vi "RT 10Hz test 1.vi"() -> ()   [LabVIEW 2014]
uses:
  <vilib>/Platform/TimedLoop/XDataNode/timing_clust.ctl
  <vilib>/Platform/TimedLoop/XDataNode/nitl_modes.ctl
  <vilib>/Platform/TimedLoop/XDataNode/wakeup.ctl
  <vilib>/FPGAPlugInAG/cRIO-9067/niLvFpga_Open_cRIO-9067.vi
  <vilib>/Utility/error.llb/Error Cluster From Error Code.vi
  <vilib>/rvi/errors/niLvFpgaAdjustHostInterfaceError.vi
  <vilib>/FPGAPlugInAG/cRIO-9067/niLvFpga_Close_cRIO-9067.vi
  <vilib>/rvi/interface/nirviOpenFPGA/nirviOpenFPGA.xnode
  FPGA Bitfiles/MAXCAT_FPGATarget5_FPGAmainv06_iLwI+xiZeAU.lvbitx
  FPGA main v06.vi
  <vilib>/Platform/TimedLoop/XDataNode/XDataNode.xnode
  <vilib>/rvi/interface/nirviReadWriteControl/nirviReadWriteControl.xnode
  <vilib>/rvi/interface/nirviCloseFPGA/nirviCloseFPGA.xnode
  NiFpgaLv.dll
  <vilib>/Platform/TimedLoop/XDataNode/XDNodeRunTimeDep.lvlib
panel:
  out "Period 2":u32
  out "Period":u32
  out "Array 1 In":fxp<+/-,35,9>[](array[numeric])
  out "Array 2 In":fxp<+/-,30,9>[](array[numeric])
  in  "stop":bool
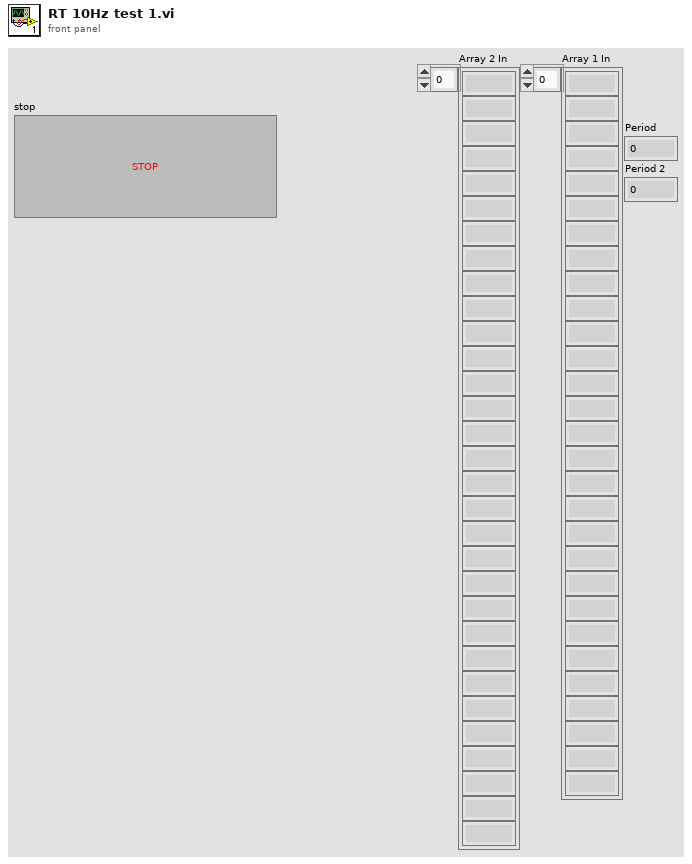
[diagram p1: front panel]
types:
  T1 = typedef "XDNodeRunTimeDep.lvlib/timing_clust.ctl" = cluster{"Expected End [f-1]":u64, "Actual End [f-1]":u64, "Finished Late? [f-1]":bool, "Expected End [i-1]":u64, "Actual End [i-1]":u64, "Finished Late? [i-1]":bool, "Expected Start [i]":u64, "Actual Start [i]":u64, "Expected Start [f]":u64, "Actual Start [f]":u64, "Source Name":string, "Structure Name":string, "Period":i64, "Deadline":i64, "Offset":i64, "Start":i64, "Priority":i32, "Timeout":i32, "Mode":T2, "Wakeup Reason":T3, "Error":errorcluster, "Source Type":string, "Secondary Source Type":string, "Global End Time":u64, "Global Start Time":u64, "Frame Duration":u64, "Iteration Duration":u64, "Assigned CPU":i32, "I/O Scan Engine Mode":u32}
  T2 = typedef "XDNodeRunTimeDep.lvlib/nitl_modes.ctl" = enum32{"No Change", "Process missed periods, maintain original phase", "Discard missed periods, maintain original phase", "Process missed periods, ignore original phase", "Discard missed periods, ignore original phase"}
  T3 = typedef "XDNodeRunTimeDep.lvlib/wakeup.ctl" = enum32{"Normal", "Aborted", "Asynchronous wakeup", "Timing source error", "Timed loop error", "Timeout"}
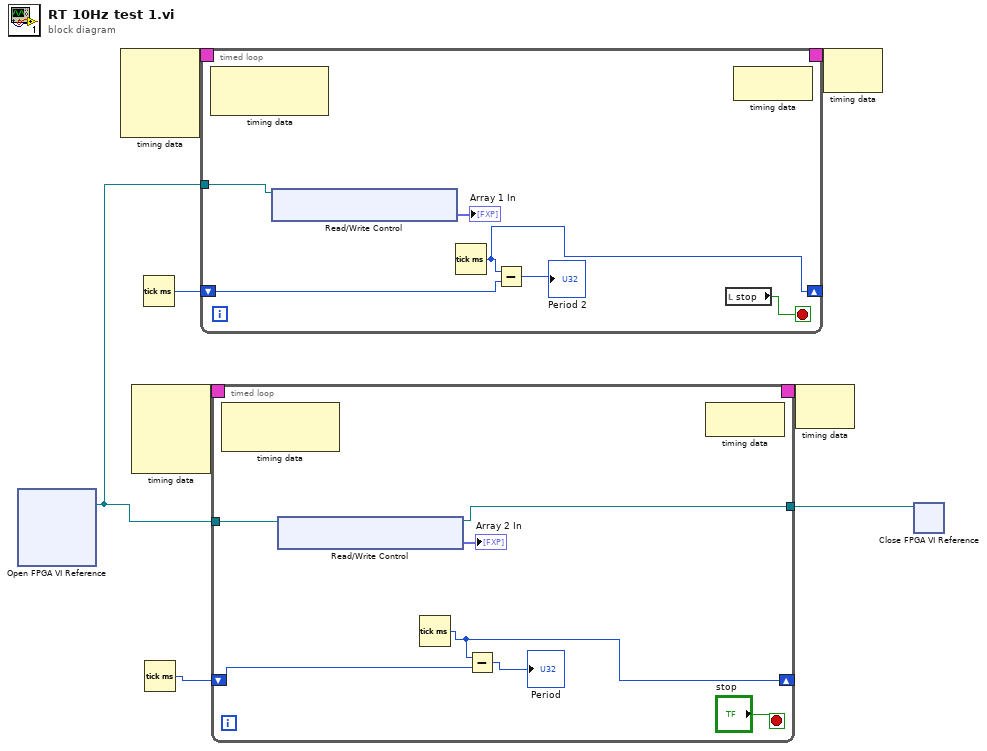
[diagram p0: block diagram]
diagram:
  n1 = xnode "Open FPGA VI Reference"() -> ("FPGA VI Reference Out"=w3:refnum<k20>)  [unwired: 2 in, 1 out]
  n2 = node-c288() -> (w5:T1)  [unwired: 4 in]
  n3 = node-c288() -> (w7:T1)  [unwired: 4 in]
  n4 = Tick Count (ms)() -> (millisecond timer value=w2:u32)
  n5 = Tick Count (ms)() -> (millisecond timer value=w1:u32)
  n6 = timed-loop {
    timing: w5 -> [_]
    timing-out: [_] -> w4
    tunnel: w3 -> [w14]
    shift-right: [w9] -> _
    shift-left: w2 -> [w11]
    stop <- w12 stop-if-true
    n7 = node-c288() -> ()  [unwired: 1 in, 2 out]
    n8 = xnode "Read/Write Control"("FPGA VI Reference In"=w14) -> ("Array 1 In"=→"Array 1 In":fxp<+/-,35,9>[])  [unwired: 1 in, 2 out]
    n9 = Tick Count (ms)() -> (millisecond timer value=w9:u32)
    n10 = Subtract(x=w9, y=w11) -> (x-y=→"Period 2":u32)
    n11 = local read "stop"() -> (w12:bool)
    n12 = node-c288() -> ()  [unwired: 1 in, 1 out]
  }
  n13 = timed-loop {
    tunnel: w3 -> [w22]
    tunnel: [w21] -> w8
    timing: w7 -> [_]
    timing-out: [_] -> w6
    shift-right: [w18] -> _
    shift-left: w1 -> [w19]
    stop <- "stop" stop-if-true
    n14 = node-c288() -> ()  [unwired: 1 in, 2 out]
    n15 = xnode "Read/Write Control"("FPGA VI Reference In"=w22) -> ("FPGA VI Reference Out"=w21:refnum<k20>, "Array 2 In"=→"Array 2 In":fxp<+/-,30,9>[])  [unwired: 1 in, 1 out]
    n16 = Tick Count (ms)() -> (millisecond timer value=w18:u32)
    n17 = Subtract(x=w18, y=w19) -> (x-y=→"Period":u32)
    n18 = node-c288() -> ()  [unwired: 1 in, 1 out]
  }
  n19 = node-c288(w6) -> ()  [unwired: 1 out]
  n20 = node-c288(w4) -> ()  [unwired: 1 out]
  n21 = xnode "Close FPGA VI Reference"("FPGA VI Reference In"=w8) -> ()  [unwired: 1 in, 1 out]
